vi "pressure-tdms-file-explorer.vi"() -> ()   [LabVIEW 2015]
panel:
  in  "stop":bool
  out "Waveform Graph":waveform(dbl)[](graph)
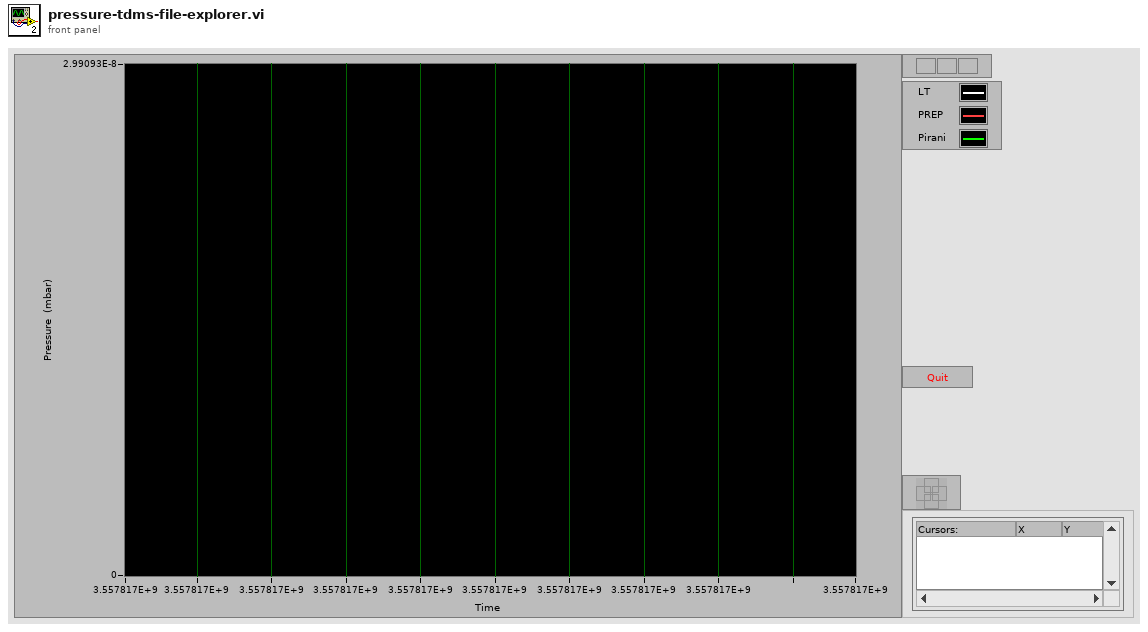
[diagram p1: front panel]
types:
  T1 = enum16{"open", "open or create", "create or replace", "create", "open (read-only)"}
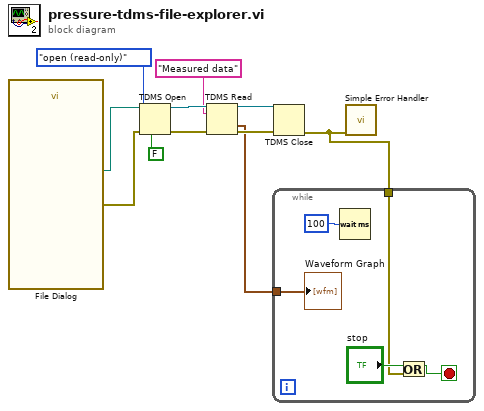
[diagram p0: block diagram]
diagram:
  n1 = call "File Dialog"() -> ("selected path"=w9:path, "error out"=w8:errorcluster)  [unwired: 12 in, 2 out]
  n2 = TDMS Open(6:FALSE ("disable buffering? (T)"), 8:w8, 10:T1."open (read-only)" ("operation (0:open)"), 11:w9) -> (0:w10:errorcluster, 3:w11:refnum<k34>)  [unwired: 3 in]
  n3 = TDMS Read(0:w11, 5:"Measured data" ("group name in"), 11:w10) -> (4:w6:refnum<k34>, 10:w5:waveform(dbl)[], 15:w7:errorcluster)  [unwired: 5 in, 3 out]
  n4 = TDMS Close(8:w7, 11:w6) -> (0:w4:errorcluster)  [unwired: 1 out]
  n5 = while {
    tunnel: w5 -> [w14]
    tunnel: w4 -> [w12]
    stop <- w13 stop-if-true
    n6 = Wait (ms)(milliseconds to wait=u32 100) -> ()  [unwired: 1 out]
    n7 = Or(x="stop", y=w12) -> (x .or. y?=w13:bool)
    "Waveform Graph" <- w14
  }
  n8 = call <vilib>:"Simple Error Handler.vi"("error in (no error)"=w4) -> ()  [unwired: 4 in, 5 out]
